vi "Z900_navX_Internal_ProcessingLoop_HandleNotifier.vi"(6 "timeout in ms (1)":i32=1, 7 "Interface TypeDefs":T1 {"I2CDevRef"."Device Address" format="%.0x"}, 8 "error in (no error)":errorcluster, 9 "Connected":bool, 10 "Registry":u8[](array[numeric]), 11 "navX Device":T7={"Interface"={"Protocol"=enum."SERIAL", "Update Rate (4Hz-100Hz)"=4, "navX Open TypeDef"=variant}, "Notify Packet"=refnum, "Loop VI Refnum"=refnum, "Ready to Close Occurrence Refnum"=refnum} {"Interface"."Update Rate (4Hz-100Hz)" min=4 max=60 step=1}) -> (0 "error out":errorcluster, 1 "Halt":bool, 2 "Registry":u8[](array[numeric]), 3 "navX Device":T7={"Interface"={"Protocol"=enum."SERIAL", "Update Rate (4Hz-100Hz)"=4, "navX Open TypeDef"=variant}, "Notify Packet"=refnum, "Loop VI Refnum"=refnum, "Ready to Close Occurrence Refnum"=refnum} {"Interface"."Update Rate (4Hz-100Hz)" min=4 max=60 step=1}, 5 "Interface TypeDefs":T1 {"I2CDevRef"."Device Address" format="%.0x"})   [LabVIEW 2015, in "navX Library v2.lvlib"]
uses:
  navX Library v2.lvlib
  _TypeDefs/Z900_navX_DeviceTypeDef.ctl
  _TypeDefs/Z900_navX_ProtocolTypeDef.ctl
  _TypeDefs/Z900_navX_NotifyPacketTypeDef.ctl
  _TypeDefs/Z900_navX_ActionTypeDef.ctl
  _TypeDefs/Z900_navX_InterfaceTypeDef.ctl
  <vilib>/Rock Robotics/WPI/SerialPort/WPI_SerialPortRef.ctl
  <vilib>/Rock Robotics/WPI/I2C/WPI_I2CDevRef.ctl
  <vilib>/Rock Robotics/SystemInterfaces/i2clib/i2c_bus.ctl
  <vilib>/Rock Robotics/WPI/SPI/WPI_SPIDevRef.ctl
  <vilib>/Rock Robotics/SystemInterfaces/spilib/spi_bus.ctl
  _TypeDefs/navX Open TypeDefs/Z900_navX_OpenTypeDef_Serial.ctl
  _NI WPI Serial USB/WPI_SerialPort_USB.ctl
  _TypeDefs/Z900_navX_SerialStreamTypeDef.ctl
  _TypeDefs/Z900_navX_ZeroVectorTypeDef.ctl
  SERIAL/Z900_navX_SERIAL_PacketChecksum.vi
  Z900_navX_Internal_SendIntegrationControl.vi
  _Util/Decode Protocol/Z900_navX_Util_DecodeProtocol_UInt16.vi
  _Util/Z900_navX_Util_LittleEndian_to_BigEndian.vi
  <vilib>/Rock Robotics/WPI/SerialPort/WPI_SerialPortReset.vi
  <vilib>/Rock Robotics/WPI/SerialPort/WPI_SerialPortWrite.vi
  <vilib>/Rock Robotics/WPI/SerialPort/WPI_SerialPortFlush.vi
  <vilib>/Rock Robotics/WPI/I2C/WPI_I2CWrite.vi
  SPI/Z900_navX_SPI_CRC.vi
  <vilib>/Rock Robotics/WPI/SPI/WPI_SPIWrite.vi
  _NI WPI Serial USB/_NI WPI Serial USB.lvlib
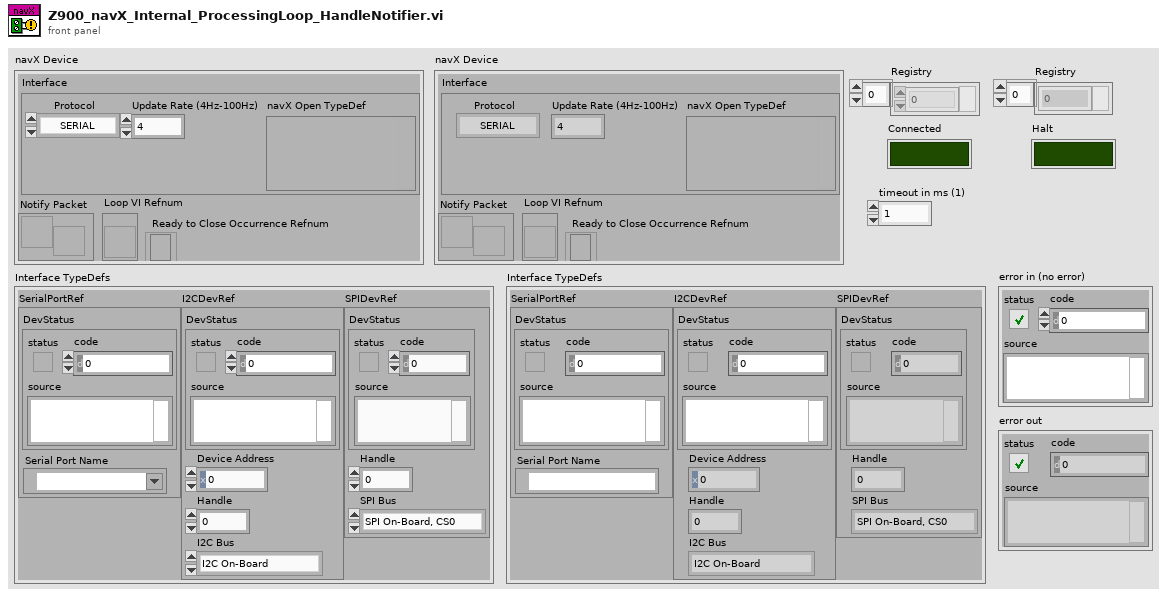
[diagram p1: front panel]
types:
  T1 = typedef "navX Library v2.lvlib/Z900_navX_InterfaceTypeDef.ctl" = cluster{"SerialPortRef":T2, "I2CDevRef":T3, "SPIDevRef":T5}
  T2 = typedef "WPI_SerialPortRef.ctl" = cluster{"DevStatus":errorcluster, "Serial Port Name":refnum<visa-resource-name>}
  T3 = typedef "WPI_I2CDevRef.ctl" = cluster{"DevStatus":errorcluster, "Device Address":u8, "Handle":i32, "I2C Bus":T4}
  T4 = typedef "i2c_bus.ctl" = enum16{"I2C On-Board", "I2C MXP", "Invalid"}
  T5 = typedef "WPI_SPIDevRef.ctl" = cluster{"DevStatus":errorcluster, "Handle":i32, "SPI Bus":T6}
  T6 = typedef "spi_bus.ctl" = enum16{"SPI On-Board, CS0", "SPI On-Board, CS1", "SPI On-Board, CS2", "SPI On-Board, CS3", "SPI MXP", "Invalid"}
  T7 = typedef "navX Library v2.lvlib/Z900_navX_DeviceTypeDef.ctl" = cluster{"Interface":cluster{"Protocol":T8, "Update Rate (4Hz-100Hz)":u8, "navX Open TypeDef":variant}, "Notify Packet":refnum<notifier>, "Loop VI Refnum":refnum<vi>, "Ready to Close Occurrence Refnum":refnum<k4>}
  T8 = typedef "navX Library v2.lvlib/Z900_navX_ProtocolTypeDef.ctl" = enum16{"SERIAL", "I2C", "SPI"}
  T9 = typedef "navX Library v2.lvlib/Z900_navX_NotifyPacketTypeDef.ctl" = cluster{"navX Action":T10, "Data":variant}
  T10 = typedef "navX Library v2.lvlib/Z900_navX_ActionTypeDef.ctl" = enum16{"None", "Halt", "Update Serial Protocol", "Zero-Yaw", "Zero-Displacement", "Zero-Velocity"}
  T11 = typedef "navX Library v2.lvlib/Z900_navX_OpenTypeDef_Serial.ctl" = cluster{"Serial Port":T12, "Stream Type":T13}
  T12 = typedef "_NI WPI Serial USB.lvlib/WPI_SerialPort_USB.ctl" = enum16{"Onboard RS-232", "MXP TTL", "USB"}
  T13 = typedef "navX Library v2.lvlib/Z900_navX_SerialStreamTypeDef.ctl" = enum16{"YRPH", "Quaterinons", "Gyro/Raw", "AHRS", "AHRSAndPositioning"}
  T14 = typedef "navX Library v2.lvlib/Z900_navX_ZeroVectorTypeDef.ctl" = cluster{"X":bool, "Y":bool, "Z":bool}
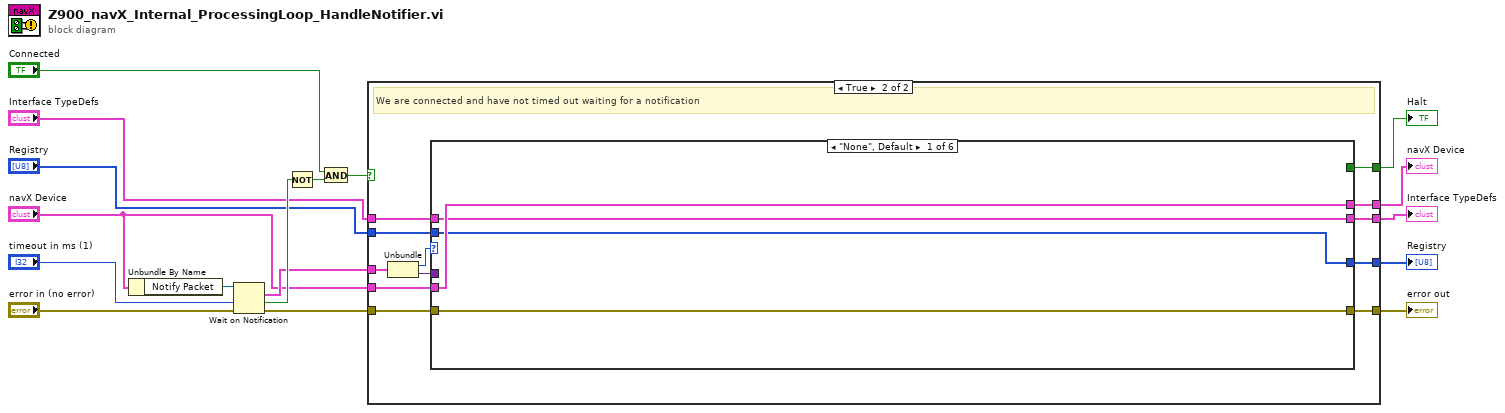
[diagram p0: block diagram]
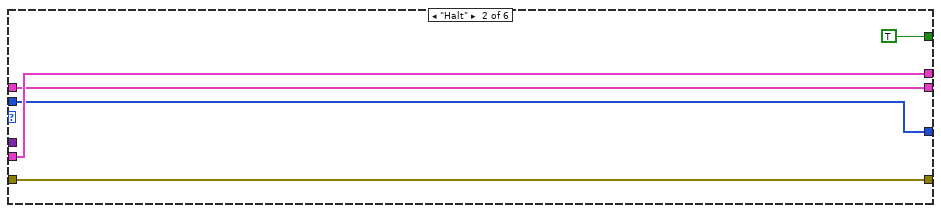
[diagram p3: hidden frame]
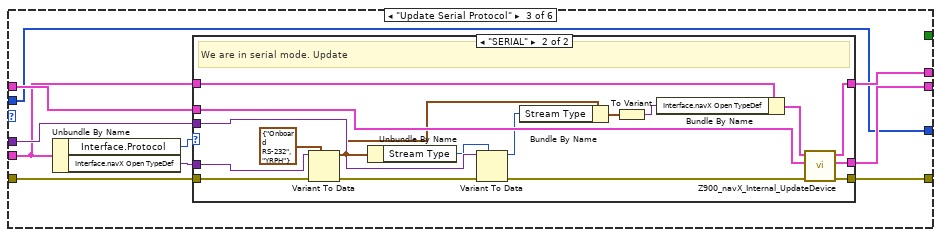
[diagram p4: hidden frame]
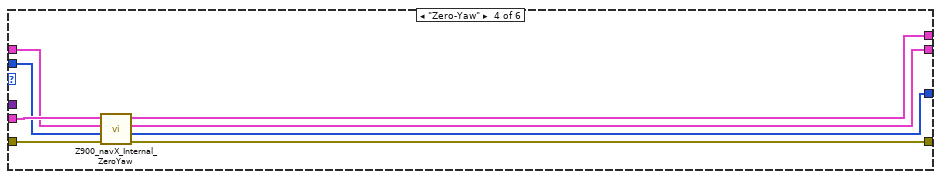
[diagram p6: hidden frame]
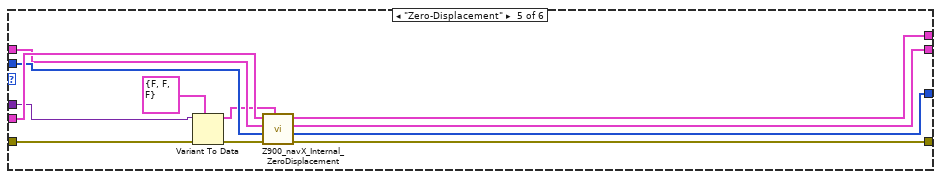
[diagram p7: hidden frame]
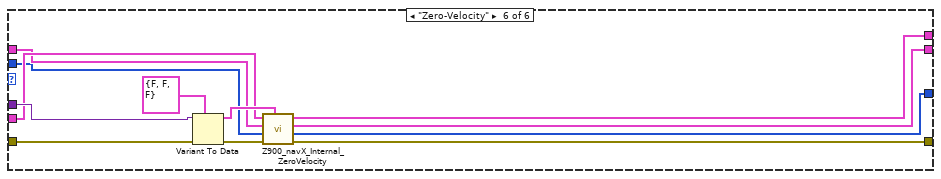
[diagram p8: hidden frame]
diagram:
  n1 = Unbundle By Name("navX Device") -> ("Notify Packet"=w16:refnum<notifier>)
  n2 = Wait on Notification(notifier=w16, timeout in ms (-1)="timeout in ms (1)", error in (no error)="error in (no error)") -> (notification=w10:T9, timed out?=w13:bool, error out=w7:errorcluster)  [unwired: 1 in, 1 out]
  n3 = Not(x=w13) -> (.not. x?=w15:bool)
  n4 = And(x="Connected", y=w15) -> (x .and. y?=w12:bool)
  n5 = case shown="True" w12 {
    tunnel: w10 -> [_ w33]
    tunnel: "navX Device" -> [w21 w31]
    tunnel: "Interface TypeDefs" -> [w20 w30]
    tunnel: [w20 w29] -> w1
    tunnel: [w21 w28] -> w2
    tunnel: w7 -> [w18 w26]
    tunnel: "Registry" -> [w19 w25]
    tunnel: [w19 w24] -> w4
    tunnel: [w18 w23] -> w6
    tunnel: [_ w22] -> w3
    frame False {
      # "We are either not connected or have timed out waiting for a notification"
    }
    frame True {
      # "We are connected and have not timed out waiting for a notification"
      n6 = Unbundle(w33) -> ("navX Action"=w32:T10, "Data"=w27:variant)
      n7 = case shown="\"None\", Default" w32 {
        tunnel: w31 -> [w37 w42 w46 w80 w92 w99]
        tunnel: w30 -> [w36 w41 w52 w78 w90 w98]
        tunnel: [w36 w41 w51 w77 w88 w95] -> w29
        tunnel: [w37 w42 w50 w79 w89 w96] -> w28
        tunnel: w27 -> [_ _ w49 _ w85 w102]
        tunnel: w26 -> [w34 w39 w47 w76 w82 w103]
        tunnel: w25 -> [w35 w40 w45 w75 w91 w97]
        tunnel: [w35 w40 w45 w74 w87 w94] -> w24
        tunnel: [w34 w39 w44 w73 w86 w93] -> w23
        tunnel: [_ TRUE _ _ _ _] -> w22
        frame "None", Default {
        }
        frame "Halt" {
        }
        frame "Update Serial Protocol" {
          n8 = Unbundle By Name(w46) -> ("Interface.Protocol"=w43:T8, "Interface.navX Open TypeDef"=w48:variant)
          n9 = case shown="\"SERIAL\"" w43 {
            tunnel: w52 -> [w54 w72]
            tunnel: [w54 w71] -> w51
            tunnel: [w55 w70] -> w50
            tunnel: w49 -> [_ w69]
            tunnel: w48 -> [_ w66]
            tunnel: w47 -> [w53 w63]
            tunnel: w46 -> [w55 w62]
            tunnel: [w53 w56] -> w44
            frame Default {
              # "We don't care if we are not in serial mode."
            }
            frame "SERIAL" {
              # "We are in serial mode. Update"
              n10 = Variant To Data(error in=w63, type=T11 {"Serial Port"=enum."Onboard RS-232", "Stream Type"=enum."YRPH"} ("navX Serial Open"), Variant=w66) -> (data=w59:T11, error out=w64:errorcluster)
              n11 = Unbundle By Name(w59) -> ("Stream Type"=w58:T13)
              n12 = Variant To Data(error in=w64, type=w58, Variant=w69) -> (data=w57:T13, error out=w68:errorcluster)
              n13 = Bundle By Name(cluster=w59, "Stream Type"=w57) -> (w67:T11)
              n14 = To Variant(anything=w67) -> (Variant=w61:variant)
              n15 = Bundle By Name(cluster=w62, "Interface.navX Open TypeDef"=w61) -> (w60:T7)
              n16 = call "Z900_navX_Internal_UpdateDevice.vi"("error in (no error)"=w68, "Interface TypeDefs"=w72, "navX Device"=w60) -> ("error out"=w56:errorcluster, "Interface TypeDefs"=w71:T1, "navX Device"=w70:T7)  [unwired: 6 in]
            }
          }
        }
        frame "Zero-Yaw" {
          n17 = call "Z900_navX_Internal_ZeroYaw.vi"("error in (no error)"=w76, "Registry"=w75, "Interface TypeDefs"=w78, "navX Device"=w80) -> ("error out"=w73:errorcluster, "Registry"=w74:u8[], "Interface TypeDefs"=w77:T1, "navX Device"=w79:T7)  [unwired: 4 in]
        }
        frame "Zero-Displacement" {
          n18 = Variant To Data(error in=w82, type=T14 {"X"=FALSE, "Y"=FALSE, "Z"=FALSE} ("Zero Vector"), Variant=w85) -> (data=w83:T14, error out=w81:errorcluster)
          n19 = call "Z900_navX_Internal_ZeroDisplacement.vi"("Zero Vector"=w83, "error in (no error)"=w81, "Registry"=w91, "Interface TypeDefs"=w90, "navX Device"=w92) -> ("error out"=w86:errorcluster, "Registry"=w87:u8[], "Interface TypeDefs"=w88:T1, "navX Device"=w89:T7)  [unwired: 3 in]
        }
        frame "Zero-Velocity" {
          n20 = Variant To Data(error in=w103, type=T14 {"X"=FALSE, "Y"=FALSE, "Z"=FALSE} ("Zero Vector"), Variant=w102) -> (data=w101:T14, error out=w100:errorcluster)
          n21 = call "Z900_navX_Internal_ZeroVelocity.vi"("Zero Vector"=w101, "error in (no error)"=w100, "Registry"=w97, "Interface TypeDefs"=w98, "navX Device"=w99) -> ("error out"=w93:errorcluster, "Registry"=w94:u8[], "Interface TypeDefs"=w95:T1, "navX Device"=w96:T7)  [unwired: 3 in]
        }
      }
    }
  }
  "error out" <- w6
  "Registry" <- w4
  "Halt" <- w3
  "Interface TypeDefs" <- w1
  "navX Device" <- w2
